vi "8.3.-Momento Invariante de Hu Normalizado - Npq.vi"(1 "q":dbl, 2 "p":dbl, 3 "Upq/u00":dbl[](array[numeric])) -> (0 "Npq":dbl)   [LabVIEW 2020]
panel:
  # "Visión Artificial - Momentos Invariantes de Hu\nDiego Cervantes Rodríguez\ndicer0.com"
  # "Momento normalizado = Npq = Upq/u00^d, donde:\nd = ((p+q)/2)+1, si p+q > 1\nd = 1, si p+q <= 1"
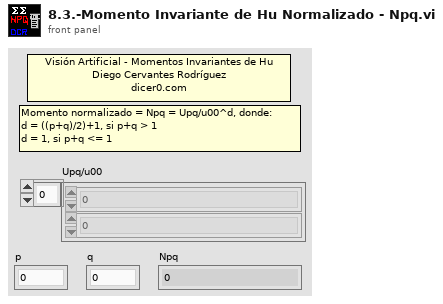
[diagram p1: front panel]
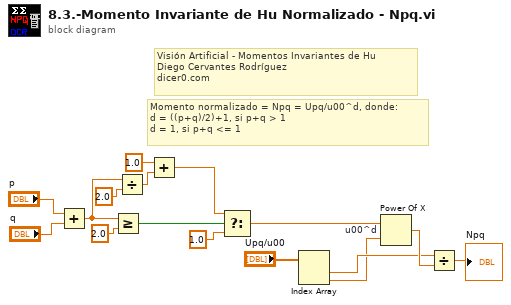
[diagram p0: block diagram]
diagram:
  # "Visión Artificial - Momentos Invariantes de Hu\nDiego Cervantes Rodríguez\ndicer0.com"
  # "Momento normalizado = Npq = Upq/u00^d, donde:\nd = ((p+q)/2)+1, si p+q > 1\nd = 1, si p+q <= 1"
  n1 = Add(x="p", y="q") -> (x+y=w11:dbl)
  n2 = Greater Or Equal?(x=w11, y=2.0) -> (x >= y?=w13:bool)
  n3 = Divide(x=w11, y=2.0) -> (x/y=w10:dbl)
  n4 = Add(x=1.0, y=w10) -> (x+y=w8:dbl)
  n5 = Select(t=w8, s=w13, f=1.0) -> (s? t:f=w7:dbl)
  n6 = Index Array "Index Array"(array="Upq/u00") -> (element #1=w4:dbl, element #2=w3:dbl)  [unwired: 2 in]
  n7 = Power Of X "u00^d"(1:w3, 2:w7) -> (0:w6:dbl)
  n8 = Divide ("u00^d")(x=w4, y=w6) -> (x/y=→"Npq":dbl)
